vi "commands.vi"(0 "Data Acq":T1=enum."NML Data Acquisition-New.vi", 1 "Scan Seq?":bool=TRUE, 3 "list com":string[](array[string]), 4 "tree com":string, 5 "option":T2) -> (2 "output":string[][](array[string]))   [LabVIEW 2020]
uses:
  Ctl/commands.ctl
  Ctl/option.ctl
  Ctl/Data Acquisition System.ctl
panel:
  out "valid":bool
  out "command":T3=enum."Comments"
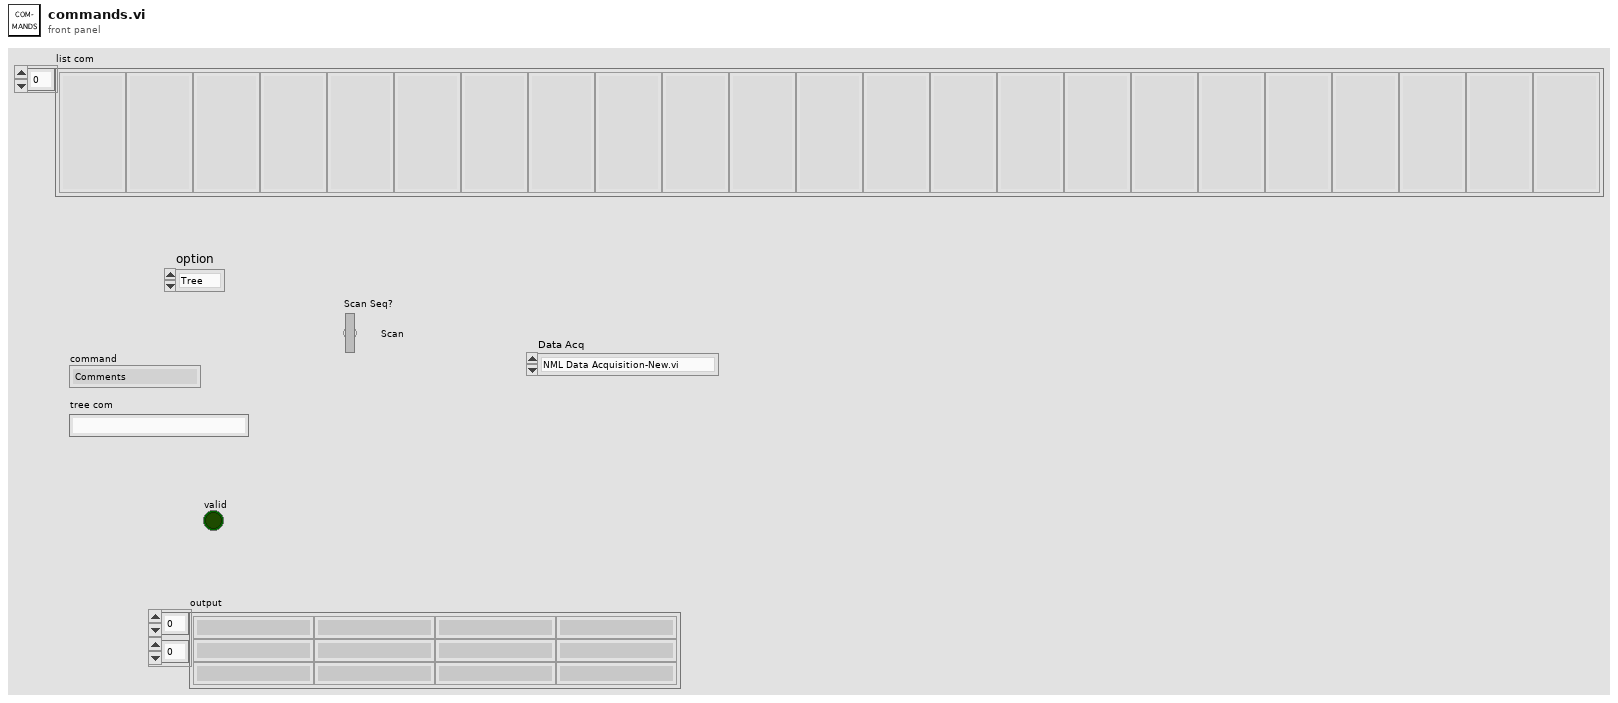
[diagram p1: front panel]
types:
  T1 = typedef "Data Acquisition System.ctl" = enum16{"NML Data Acquisition-old.vi", "NML Data Acquisition-New.vi"}
  T2 = typedef "option.ctl" = enum16{"Tree", "List"}
  T3 = typedef "commands.ctl" = enum16{"Voltage Ramp", "Many Voltage Ramp", "Current Ramp", "Many Current Ramp", "Comments", "Set Field", "Many Set Field", "Abort Sequence", "New-Stop File", "Wait(sec)", "BLM Control", "Many BLM Control", "Stepper Mover", "Many Stepper Mover", "LS336 Ramp Temp", "LakeShore Ramp", "VI Server Control", "LS370 Change Excitation", "Wait Until", "Nothing"}
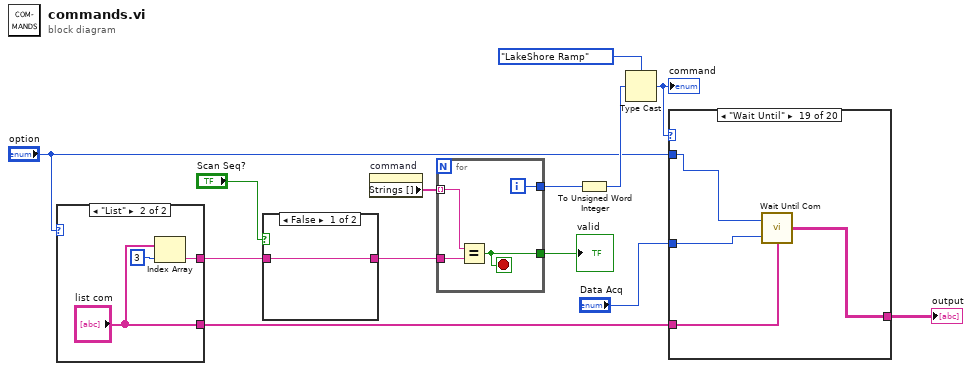
[diagram p0: block diagram]
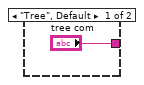
[diagram p2: hidden frame]
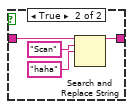
[diagram p3: hidden frame]
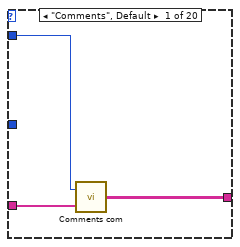
[diagram p4: hidden frame]
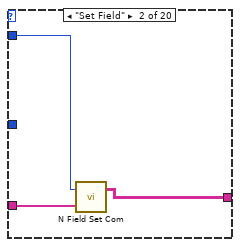
[diagram p5: hidden frame]
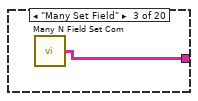
[diagram p6: hidden frame]
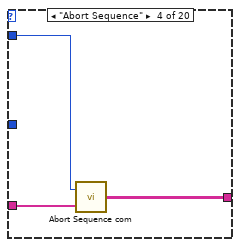
[diagram p7: hidden frame]
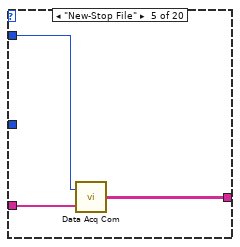
[diagram p8: hidden frame]
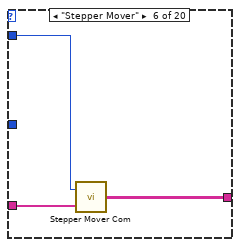
[diagram p9: hidden frame]
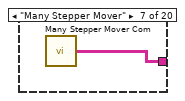
[diagram p10: hidden frame]
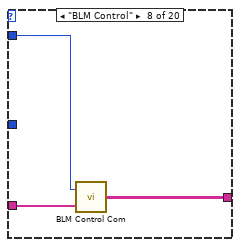
[diagram p11: hidden frame]
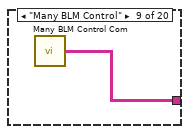
[diagram p12: hidden frame]
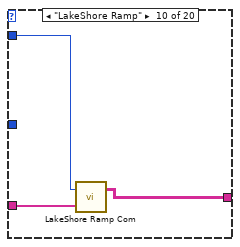
[diagram p13: hidden frame]
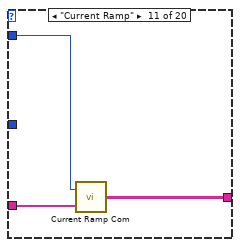
[diagram p14: hidden frame]
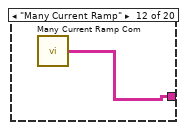
[diagram p15: hidden frame]
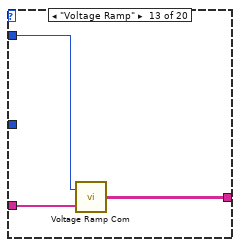
[diagram p16: hidden frame]
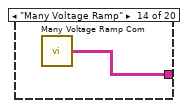
[diagram p17: hidden frame]
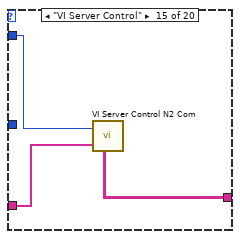
[diagram p18: hidden frame]
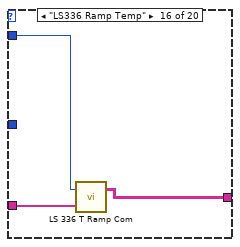
[diagram p19: hidden frame]
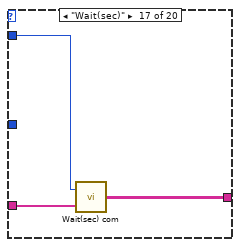
[diagram p20: hidden frame]
diagram:
  n1 = case shown="\"List\"" "option" {
    tunnel: ["tree com" w16] -> w3
    tunnel: [_ "list com"] -> w2
    frame "Tree", Default {
    }
    frame "List" {
      n2 = Index Array(array="list com", index=3 ("disabled index (col)")) -> (element=w16:string)
    }
  }
  n3 = case shown="False" "Scan Seq?" {
    tunnel: w3 -> [w18 w20]
    tunnel: [w18 w19] -> w5
    frame False {
    }
    frame True {
      n4 = Search and Replace String(input string=w20, search string="Scan", replace string="haha" ("replace string (\"\")")) -> (result string=w19:string)  [unwired: 5 in, 3 out]
    }
  }
  n5 = property on="command" class="Enum (strict)"() -> ("Strings []"=w13:string[])  [unwired: 2 in, 2 out]
  n6 = for {
    tunnel: w13 -> [w26] mode=indexing
    tunnel: [w24] -> w8
    tunnel: [w25] -> w12
    tunnel: w5 -> [w23]
    i -> [w24]
    stop <- w25 stop-if-true
    n7 = Equal?(x=w26, y=w23) -> (x = y?=w25:bool)
  }
  "valid" <- w12
  n8 = To Unsigned Word Integer(number=w8) -> (unsigned 16bit integer=w7:u16)
  n9 = Type Cast(type=commands."LakeShore Ramp" ("command"), x=w7) -> (*(type *) &x=w10:T3)
  "command" <- w10
  n10 = case shown="\"Wait Until\"" w10 {
    tunnel: [w29 w30 w33 w36 w37 w40 w43 w44 w47 w48 w51 w54 w55 w58 w60 w62 w67 w70 w71 _] -> w9
    tunnel: "option" -> [w28 w32 _ w35 w39 w42 _ w46 _ w50 w53 _ w57 _ w59 w63 w66 w69 w74 _]
    tunnel: w2 -> [w27 w31 _ w34 w38 w41 _ w45 _ w49 w52 _ w56 _ w61 w64 w65 w68 w72 _]
    tunnel: "Data Acq" -> [_ _ _ _ _ _ _ _ _ _ _ _ _ _ _ _ _ _ w73 _]
    frame "Comments", Default {
      n11 = call "Comments com.vi"("command text in"=w27, "option"=w28) -> ("Command text out"=w29:string[][])
    }
    frame "Set Field" {
      n12 = call "N Field Set Com.vi"("command text in"=w31, "option"=w32) -> ("Command text out"=w30:string[][])  [unwired: 1 in]
    }
    frame "Many Set Field" {
      n13 = call "Many N Field Set Com.vi"() -> ("Command text"=w33:string[][])
    }
    frame "Abort Sequence" {
      n14 = call "Abort Sequence com.vi"("command text in"=w34, "option"=w35) -> ("Command text out"=w36:string[][])
    }
    frame "New-Stop File" {
      n15 = call "Data Acq Com.vi"("command text in"=w38, "option"=w39) -> ("Command text out"=w37:string[][])
    }
    frame "Stepper Mover" {
      n16 = call "Stepper Mover Com.vi"("command text in"=w41, "option"=w42) -> ("Command text out"=w40:string[][])
    }
    frame "Many Stepper Mover" {
      n17 = call "Many Stepper Mover Com.vi"() -> ("Command text"=w43:string[][])
    }
    frame "BLM Control" {
      n18 = call "BLM Control Com.vi"("command text in"=w45, "option"=w46) -> ("Command text out"=w44:string[][])
    }
    frame "Many BLM Control" {
      n19 = call "Many BLM Control Com.vi"() -> ("Command text"=w47:string[][])
    }
    frame "LakeShore Ramp" {
      n20 = call "LakeShore Ramp Com.vi"("command text in"=w49, "option"=w50) -> ("Command text out"=w48:string[][])  [unwired: 1 in]
    }
    frame "Current Ramp" {
      n21 = call "Current Ramp Com.vi"("command text in"=w52, "option"=w53) -> ("Command text out"=w51:string[][])
    }
    frame "Many Current Ramp" {
      n22 = call "Many Current Ramp Com.vi"() -> ("Command text"=w54:string[][])  [unwired: 1 in]
    }
    frame "Voltage Ramp" {
      n23 = call "Voltage Ramp Com.vi"("command text in"=w56, "option"=w57) -> ("Command text out"=w55:string[][])
    }
    frame "Many Voltage Ramp" {
      n24 = call "Many Voltage Ramp Com.vi"() -> ("Command text"=w58:string[][])
    }
    frame "VI Server Control" {
      n25 = call "VI Server Control N2 Com.vi"("command text in"=w61, "option"=w59) -> ("Command text out"=w60:string[][])
    }
    frame "LS336 Ramp Temp" {
      n26 = call "LS 336 T Ramp Com.vi"("command text in"=w64, "option"=w63) -> ("Command text out"=w62:string[][])  [unwired: 1 in]
    }
    frame "Wait(sec)" {
      n27 = call "Wait(sec) com.vi"("command text in"=w65, "option"=w66) -> ("Command text out"=w67:string[][])
    }
    frame "LS370 Change Excitation" {
      n28 = call "LS370 Change Excitation Com.vi"("command text in"=w68, "option"=w69) -> ("Command text out"=w70:string[][])
    }
    frame "Wait Until" {
      n29 = call "Wait Until Com.vi"("command text in"=w72, "Data Acq"=w73, "option"=w74) -> ("Command text out"=w71:string[][])
    }
    frame "Nothing" {
    }
  }
  "output" <- w9
